vi "Add Transfer Group with Children.vi"(6 "Plugin Decimation (1)":u64=1, 7 "Transfer Group configuration":T1={"name"="", "direction"=enum."Tx", "cycle timing"={"priority"=0, "decimation"=1, "offset"=0}, "thread index"=-1, "settings"=[], "Transfers"=[], "timeout behavior"=enum."Increment Late Count"} {"Transfers"."channels"."string offset" format="%d bytes"}, 8 "error in (no error)":errorcluster, 9 "Transfer Group":refnum<class "Transfer Group.lvclass">, 10 "parent tag":string, 11 "Application Data In":T10) -> (0 "error out":errorcluster, 2 "average bandwidth":dbl format="%.0g bytes", 3 "Application Data In":T10)   [LabVIEW 2017, in "DSF Core.lvlib"]
uses:
  DSF Core.lvlib
  Main VI/Application Data.ctl
  LabVIEW-Memory/Source/Classes/Pointer/Pointer.lvclass
  Classes/Framework/Framework.lvclass
  Buffer Reader/Buffer Data.ctl
  Classes/Buffer/Buffer.lvclass
  C:/Git/DSF/LabVIEW-Memory/Source/Classes/Pointer/Pointer.lvclass
  Classes/Transfer Group Status/Status.lvclass
  Typedefs/DSF Data Type.ctl
  Typedefs/DSF Engine Channel Configuration.ctl
  Typedefs/DSF Settings Info.ctl
  Typedefs/DSF Byte Order.ctl
  Typedefs/DSF Engine Framework Configuration.ctl
  Typedefs/DSF Engine Plugin Configuration.ctl
  Typedefs/DSF Timing Info.ctl
  Typedefs/DSF Engine Plugin Thread Configuration.ctl
  Typedefs/DSF Engine Transfer Group Configuration.ctl
  Typedefs/DSF Direction.ctl
  Typedefs/DSF Engine Transfer Configuration.ctl
  Typedefs/DSF Timeout Behavior.ctl
  Classes/Transfer Group/Transfer Group.lvclass
  Classes/Transfer Group/Transfer Group.lvclass/Transfer Group.ctl
  Classes/Buffers/Buffers.lvclass/Buffers.ctl
  Classes/Timing/Timing.lvclass/Timing.ctl
  ID to Tree Items/Tree Item Type.ctl
  Classes/Transfer/Transfer.lvclass/Transfer.ctl
  Add Buffers with Children.vi
  Classes/Buffer/Get Buffer Size.vi
  Classes/Buffers/Get Inline Buffer.vi
  Classes/Buffers/Get Async Buffer.vi
  Add Buffer Channels.vi
  Sizeof.vi
  LabVIEW-Memory/Source/Classes/Pointer/Get Size.vi
  Classes/Buffer/Subset Buffer.vi
  Classes/Timing/Timing.lvclass
  Classes/Buffers/Buffers.lvclass
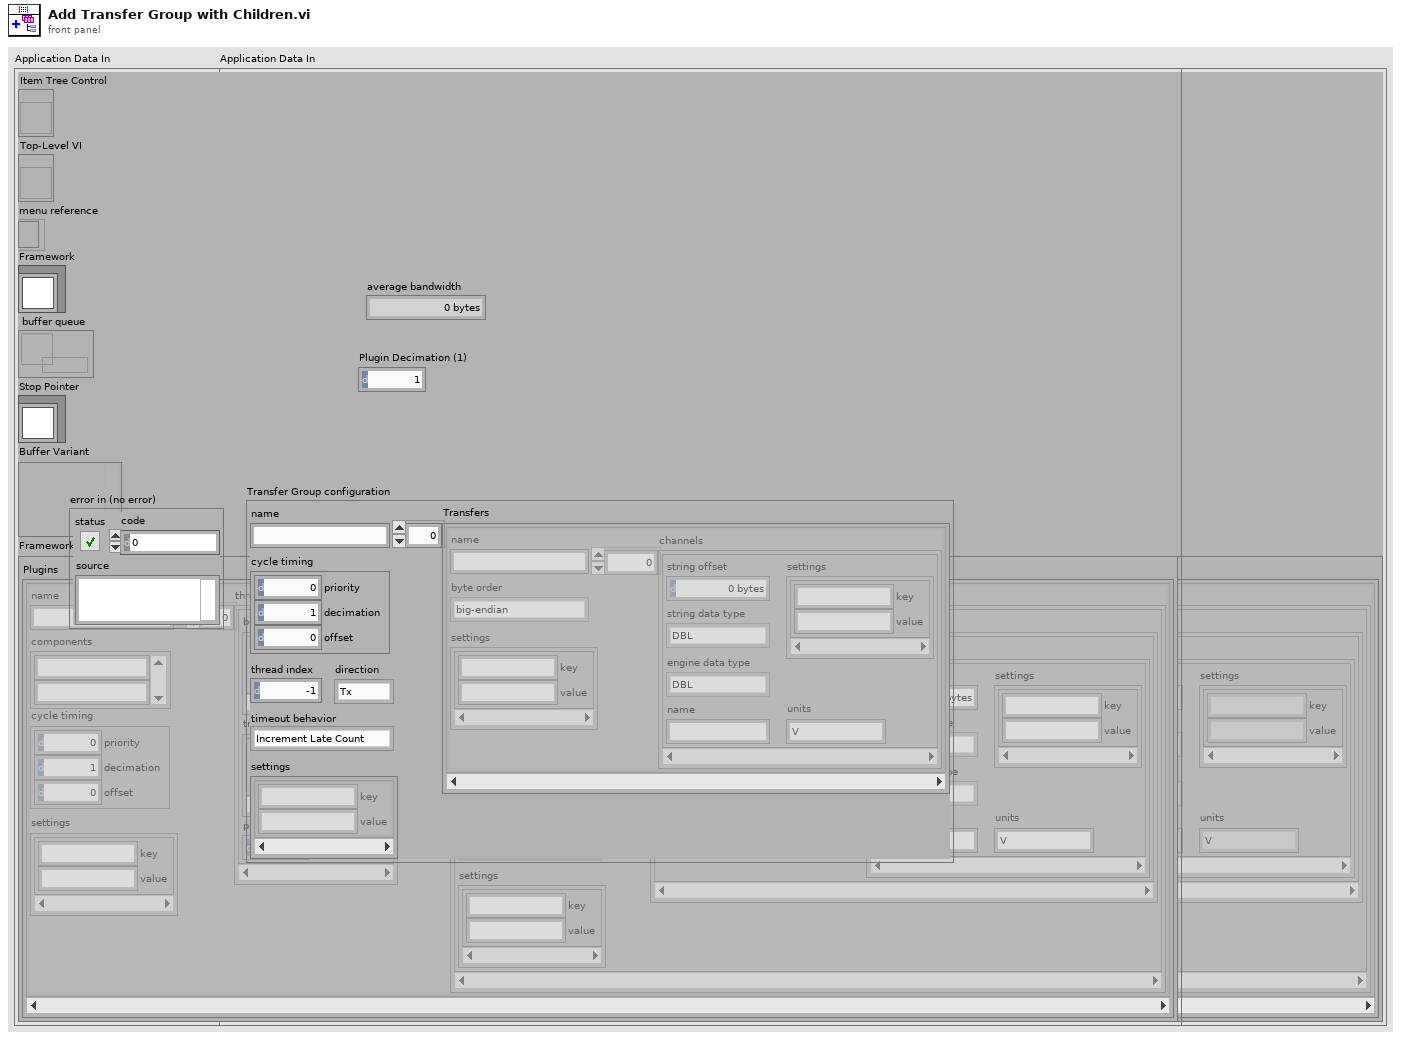
[diagram p1: front panel]
types:
  T1 = typedef "DSF Core.lvlib/DSF Engine Transfer Group Configuration.ctl" = cluster{"name":string, "direction":T2, "cycle timing":T3, "thread index":i32, "settings":T4, "Transfers":T5[], "timeout behavior":T9}
  T2 = typedef "DSF Core.lvlib/DSF Direction.ctl" = enum8{"Tx", "Rx"}
  T3 = typedef "DSF Core.lvlib/DSF Timing Info.ctl" = cluster{"priority":u64, "decimation":u64, "offset":u64}
  T4 = typedef "DSF Core.lvlib/DSF Settings Info.ctl" = cluster{"key":string, "value":string}[]
  T5 = typedef "DSF Core.lvlib/DSF Engine Transfer Configuration.ctl" = cluster{"name":string, "byte order":T6, "settings":T4, "channels":T7[]}
  T6 = typedef "DSF Core.lvlib/DSF Byte Order.ctl" = enum8{"big-endian", "little-endian"}
  T7 = typedef "DSF Core.lvlib/DSF Engine Channel Configuration.ctl" = cluster{"string offset":u64, "string data type":T8, "engine data type":T8, "name":string, "settings":T4, "units":string}
  T8 = typedef "DSF Core.lvlib/DSF Data Type.ctl" = enum8{"Bool", "SGL", "DBL", "I8", "I16", "I32", "I64", "U8", "U16", "U32", "U64"}
  T9 = typedef "DSF Core.lvlib/DSF Timeout Behavior.ctl" = enum8{"Increment Late Count", "Throw Error"}
  T10 = typedef "DSF Core.lvlib/Application Data.ctl" = cluster{"Item Tree Control":refnum<vi>, "Top-Level VI":refnum<vi>, "menu reference":refnum<k9>, "Framework":refnum<class "Framework.lvclass">, "buffer queue":refnum<queue>, "Stop Pointer":refnum<class "Pointer.lvclass">, "Buffer Variant":variant, "Framework Configuration":T11}
  T11 = typedef "DSF Core.lvlib/DSF Engine Framework Configuration.ctl" = cluster{"Plugins":T12[]}
  T12 = typedef "DSF Core.lvlib/DSF Engine Plugin Configuration.ctl" = cluster{"name":string, "components":string[], "cycle timing":T3, "threads":T13[], "Transfer Groups":T1[], "settings":T4}
  T13 = typedef "DSF Core.lvlib/DSF Engine Plugin Thread Configuration.ctl" = cluster{"buffer converter settings":T4, "transceiver settings":T4, "processor":i32, "priority offset":i16}
  T14 = typedef "DSF Core.lvlib/Buffer Data.ctl" = cluster{"Buffer":refnum<class "Buffer.lvclass">, "Status":refnum<class "Status.lvclass">, "decimation":u64, "avg bandwidth":dbl, "data type":T8, "units":string, "channels":T7[], "channel":bool, "engine (T) / string (F)":bool, "byte order":T6}
  T15 = typedef "DSF Core.lvlib/Tree Item Type.ctl" = enum16{"Framework", "Plugin Group", "Plugin", "Group", "Transfer", "Buffer", "Channel"}
  T16 = typedef "DSF Core.lvlib/Tree Item.ctl" = cluster{"Left Cell String":string, "Child Text":string[], "Child Tag":string, "Glyph Index":i32}
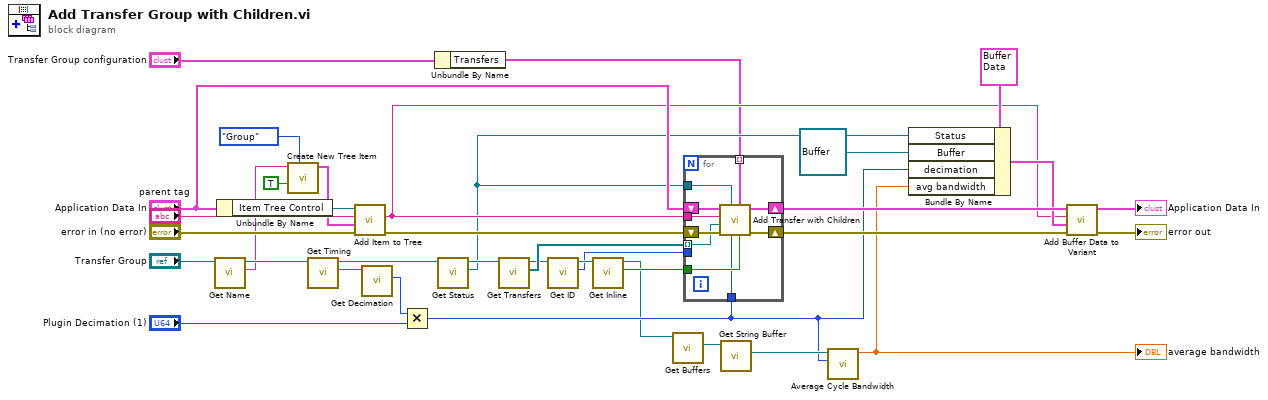
[diagram p0: block diagram]
diagram:
  n1 = call "Get Name.vi"("Transfer Group in"="Transfer Group") -> ("name"=w25:string, "Transfer Group out"=w28:refnum<class "Transfer Group.lvclass">)  [unwired: 9 in]
  n2 = Unbundle By Name("Application Data In") -> ("Item Tree Control"=w30:refnum<vi>)
  n3 = call "Create New Tree Item.vi"("Item Type"=Tree_Item_Type."Group", "found?"=TRUE, "Left Cell String"=w25) -> ("Item"=w32:T16)  [unwired: 7 in, 1 out]
  n4 = call "Get Timing.vi"("Transfer Group in"=w28) -> ("Timing"=w23:refnum<class "Timing.lvclass">, "Transfer Group out"=w16:refnum<class "Transfer Group.lvclass">)  [unwired: 9 in]
  n5 = call "Add Item to Tree.vi"("error in (no error)"="error in (no error)", "Item"=w32, "parent tag"="parent tag", "TreeControl in"=w30) -> ("error out"=w21:errorcluster, "new item tag"=w13:string)  [unwired: 5 in, 1 out]
  n6 = call "Get Decimation.vi"("Timing in"=w23) -> ("Decimation"=w27:u64)  [unwired: 9 in, 1 out]
  n7 = Multiply(x=w27, y="Plugin Decimation (1)") -> (x*y=w9:u64)
  n8 = Unbundle By Name("Transfer Group configuration") -> ("Transfers"=w2:T5[])
  n9 = call "Get Status.vi"("Transfer Group in"=w16) -> ("status pointer"=w12:refnum<class "Status.lvclass">, "Transfer Group out"=w15:refnum<class "Transfer Group.lvclass">)  [unwired: 9 in]
  n10 = call "Get Transfers.vi"("Transfer Group in"=w15) -> ("Transfers"=w31:refnum<class "Transfer.lvclass">[], "Transfer Group out"=w7:refnum<class "Transfer Group.lvclass">)  [unwired: 9 in]
  n11 = call "Get ID.vi"("Transfer Group in"=w7) -> ("id"=w4:i32, "Transfer Group out"=w5:refnum<class "Transfer Group.lvclass">)  [unwired: 9 in]
  n12 = call "Get Inline.vi"("Transfer Group in"=w5) -> ("inline"=w8:bool, "Transfer Group out"=w6:refnum<class "Transfer Group.lvclass">)  [unwired: 9 in]
  n13 = call "Get Buffers.vi"("Transfer Group in"=w6) -> ("Buffers"=w24:refnum<class "Buffers.lvclass">)  [unwired: 9 in, 1 out]
  n14 = for {
    shift-right: [w45] -> w20
    shift-left: "Application Data In" -> [w47]
    shift-right: [w44] -> w19
    shift-left: w21 -> [w46]
    tunnel: w31 -> [w43] mode=indexing
    tunnel: w13 -> [w42]
    tunnel: w8 -> [w41]
    tunnel: w9 -> [w40]
    tunnel: w12 -> [w39]
    tunnel: w4 -> [_]
    tunnel: w2 -> [w38] mode=indexing
    n15 = call "Add Transfer with Children.vi"("inline"=w41, "Transfer configuration"=w38, "Group Decimation (1)"=w40, "Transfer Group Status"=w39, "error in (no error)"=w46, "Transfer"=w43, "parent tag"=w42, "Application Data In"=w47) -> ("error out"=w44:errorcluster, "Application Data Out"=w45:T10)  [unwired: 2 in]
  }
  n16 = call "Get String Buffer.vi"("Buffers in"=w24) -> ("String Buffer"=w10:refnum<class "Buffer.lvclass">)  [unwired: 9 in, 1 out]
  n17 = call "Average Cycle Bandwidth.vi"("Decimation"=w9, "Buffer"=w10) -> ("avergage cycle bandwidth"=w11:dbl)  [unwired: 9 in]
  "average bandwidth" <- w11
  n18 = Bundle By Name(cluster=T14 {"Buffer"=refnum, "Status"=refnum, "decimation"=0, "avg bandwidth"=0.0, "data type"=enum."Bool", "units"="", "channels"=[], "channel"=FALSE, "engine (T) / string (F)"=FALSE, "byte order"=enum."little-endian"} ("Buffer data"), "Status"=w12, "Buffer"=refnum<class "Buffer.lvclass"> refnum, "decimation"=w9, "avg bandwidth"=w11) -> (w14:T14)
  n19 = call "Add Buffer Data to Variant.vi"("error in (no error)"=w19, "Buffer data"=w14, "tag"=w13, "Application Data In in"=w20) -> ("error out"=→"error out":errorcluster, "Application Data In out"=→"Application Data In":T10)  [unwired: 6 in]
